vi "OAT IIR Preprocess Filter.vi"   [LabVIEW 2017, in "SoundVib_RefDataProcess.lvlib"]
doc: "Designs an IIR filter and filters the <B>scaled signal [EU]</B>. Each instance of this VI maintains its own state; use the N Waveforms instance of this VI to process an array of channels. Wire data to the <B>scaled signal [EU]</B> input to determine the polymorphic instance to use or manually select the instance."
uses:
  <vilib>/addons/Sound and Vibration/Order Analysis/Referece Data Processing/SoundVib_RefDataProcess.lvlib
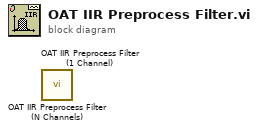
[diagram p0: block diagram]
diagram:
  n1 = call <vilib>:"OAT IIR Preprocess Filter (N Channels).vi"() -> ()  [unwired: 14 in, 2 out]
  n2 = call <vilib>:"OAT IIR Preprocess Filter (1 Channel).vi"() -> ()  [unwired: 14 in, 2 out]
